vi "Buffer read.vi"(8 "error in (no error)":errorcluster, 10 "Timeout [ms]":dbl=5000.0, 11 "VISA resource name":refnum<visa-resource-name>) -> (0 "error out":errorcluster, 2 "Received String":string, 3 "VISA resource name out":refnum<visa-resource-name>)   [LabVIEW 2017, in "RadWag balances and scales.lvlib"]
doc: "Reads data from serial port, with the usage of shift register."
uses:
  <instrlib>/Radwag Balances and Scales/Public/RadWag balances and scales.lvlib
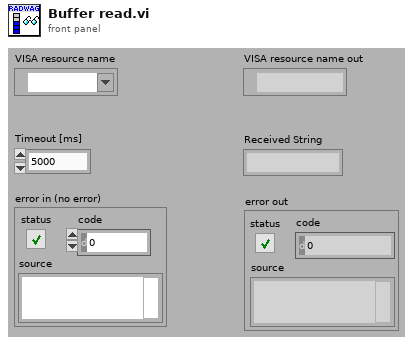
[diagram p1: front panel]
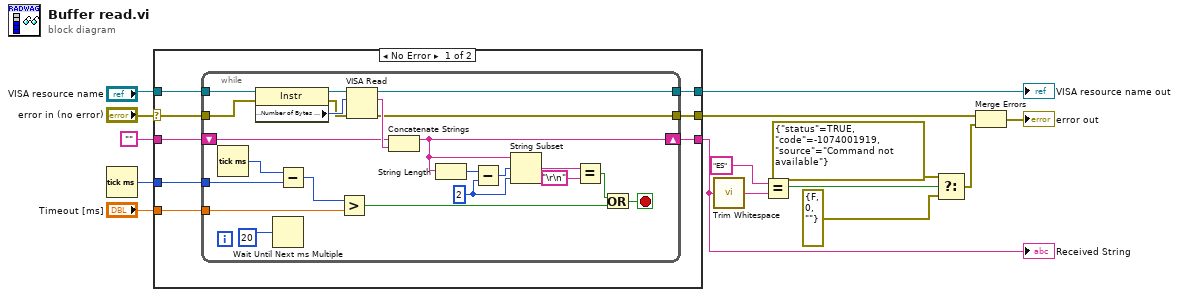
[diagram p0: block diagram]
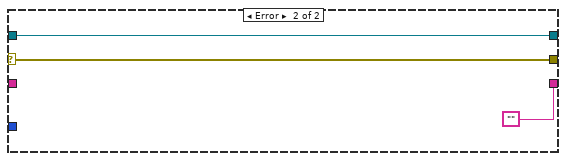
[diagram p2: hidden frame]
diagram:
  n1 = Tick Count (ms)() -> (millisecond timer value=w12:u32)
  n2 = case shown="No Error" "error in (no error)" {
    selector: "error in (no error)" -> [w16 w47]
    tunnel: [w23 ""] -> w2
    tunnel: "VISA resource name" -> [w22 w49]
    tunnel: "Timeout [ms]" -> [w21 _]
    tunnel: "" -> [w20 _]
    tunnel: w12 -> [w19 _]
    tunnel: [w18 w49] -> w11
    tunnel: [w17 w47] -> w9
    frame No Error {
      n3 = while {
        tunnel: w19 -> [w39]
        shift-right: [w31] -> w23
        shift-left: w20 -> [w45]
        tunnel: w21 -> [w37]
        tunnel: w16 -> [w35]
        tunnel: w22 -> [w36]
        tunnel: [w34] -> w17
        tunnel: [w33] -> w18
        stop <- w41 stop-if-true
        w29 = 2 ("length (rest)")
        n4 = Tick Count (ms)() -> (millisecond timer value=w40:u32)
        n5 = property class="Instr"(reference=w36, error in=w35) -> (reference out=w44:refnum<visa-resource-name>, error out=w42:errorcluster, "Serial Settings:Number of Bytes at Serial Port"=w43:u32)
        n6 = Wait Until Next ms Multiple(millisecond multiple=u32 20) -> ()  [unwired: 1 out]
        n7 = Subtract(x=w40, y=w39) -> (x-y=w38:u32)
        n8 = Greater?(x=w38, y=w37) -> (0:w24:bool)
        n9 = VISA Read(VISA resource name=w44, byte count=w43, error in (no error)=w42) -> (VISA resource name out=w33:refnum<visa-resource-name>, read buffer=w46:string, error out=w34:errorcluster)  [unwired: 1 out]
        n10 = Concatenate Strings(w45, w46) -> (w31:string)
        n11 = String Length(string=w31) -> (length=w30:i32)
        n12 = Subtract(x=w30, y=w29) -> (x-y=w26:i32)
        n13 = String Subset(string=w31, offset (0)=w26, length (rest)=w29) -> (substring=w27:string)
        n14 = Equal?(x=w27, y="\r\n") -> (x = y?=w25:bool)
        n15 = Or(x=w25, y=w24) -> (x .or. y?=w41:bool)
      }
    }
    frame Error {
    }
  }
  "VISA resource name out" <- w11
  "Received String" <- w2
  n16 = call <vilib>:"Trim Whitespace.vi"("string"=w2) -> ("trimmed string"=w1:string)  [unwired: 1 in]
  n17 = Equal?(x="ES" ("y"), y=w1) -> (x = y?=w7:bool)
  n18 = Select(t=errorcluster {"status"=TRUE, "code"=-1074001919, "source"="Command not available"} ("error in (no error)"), s=w7, f=errorcluster {"status"=FALSE, "code"=0, "source"=""} ("error constant")) -> (s? t:f=w5:errorcluster)
  n19 = Merge Errors(w9, w5) -> (→"error out":errorcluster)
